vi "Material-Line1-Aquisition.vi"(8 "error in (no error)":errorcluster, 11 "Material-RunTest in":refnum<class "Material-RunTest.lvclass">) -> (0 "error out":errorcluster, 3 "Material-RunTest out":refnum<class "Material-RunTest.lvclass">)   [LabVIEW 2013, in "Material-RunTest.lvclass"]
uses:
  Material-RunTest.lvclass
  Material-RunTest.lvclass/Material-RunTest.ctl
  <instrlib>/Keyence LK-G5000/Public/enum/LKIF_OUTNO.ctl
  <userlib>/_MGI/1D Array/MGI Average/MGI Average (SGL[]).vi
  <instrlib>/Keyence LK-G5000/Keyence LK-G5000.lvlib
  Motion Control/Motion-ControlAll.lvclass
panel:
  out "Laser Value":sgl format="%_6g"
  out "Init Meas1":dbl[](array[numeric])
  out "stop collecting":bool
  out "Meas 1 Dyn Data":dbl[](graph)
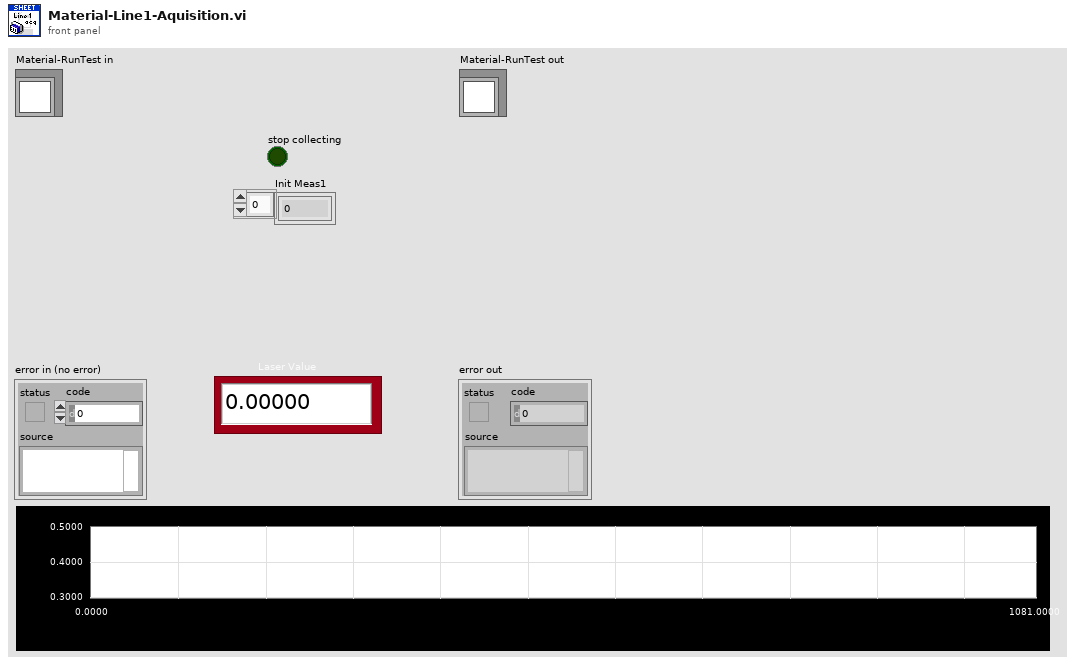
[diagram p1: front panel]
types:
  T1 = typedef "Keyence LK-G5000.lvlib/LKIF_OUTNO.ctl" = i32
  T2 = typedef "Keyence LK-G5000.lvlib/LKIF_FLOATRESULT.ctl" = i32
  T3 = cluster{"OutNo":i32, "LKIF_FLOATRESULT":T2, "Value":sgl}[]
  T4 = cluster{"OutNo":i32, "LKIF_FLOATRESULT":T2, "Value":sgl}
  T5 = cluster{waveform(dbl), waveform(dbl), waveform(dbl)}
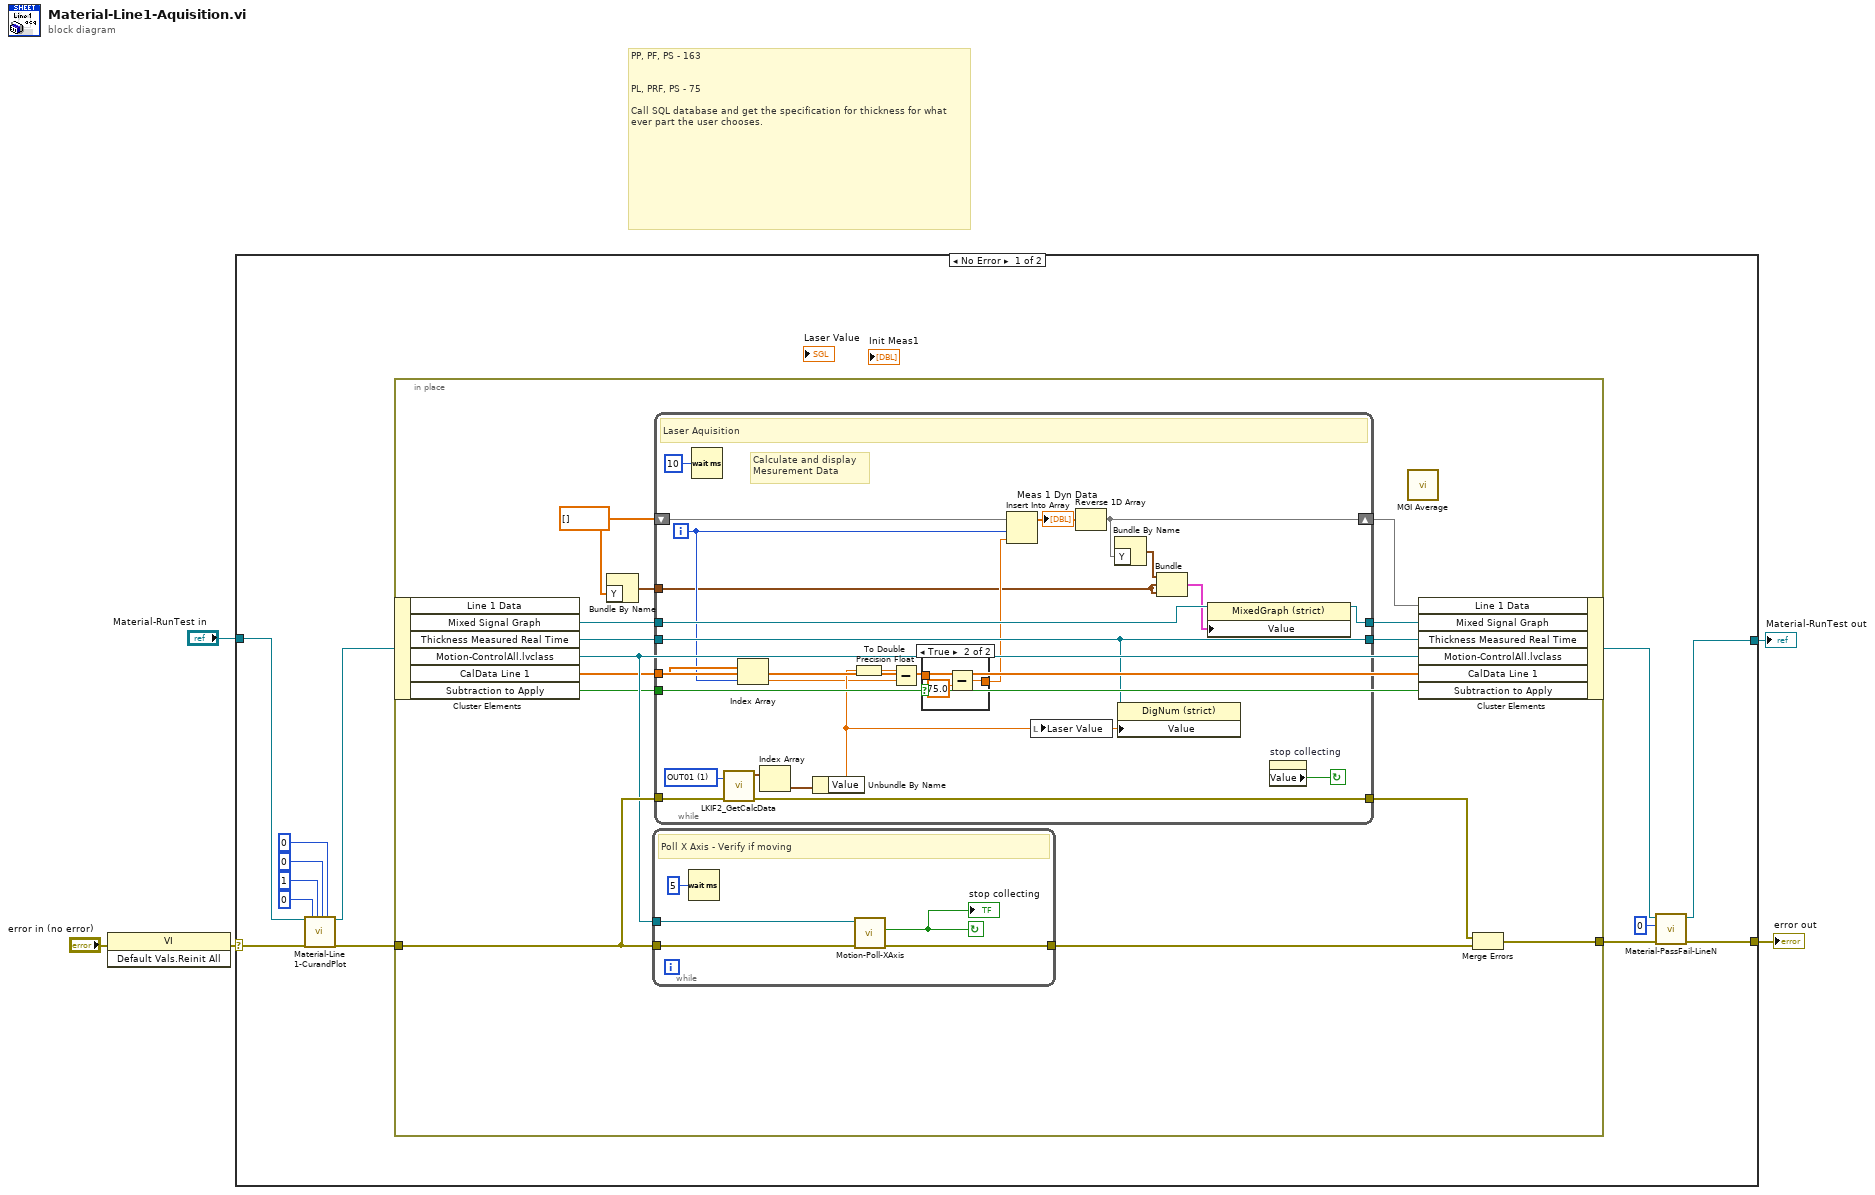
[diagram p0: block diagram]
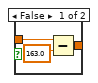
[diagram p2: hidden frame]
diagram:
  # "PP, PF, PS - 163\n\n\nPL, PRF, PS - 75\n\nCall SQL database and get the specification for thickness for what ever part the user chooses."
  n1 = invoke class="VI" method="Default Vals.Reinit All"(error in="error in (no error)") -> (error out=w1:errorcluster)  [unwired: 2 in, 2 out]
  n2 = case shown="No Error" w1 {
    selector: w1 -> [w13 w69]
    tunnel: [w6 w69] -> w5
    tunnel: [w7 w68] -> w3
    tunnel: "Material-RunTest in" -> [w18 w68]
    frame No Error {
      n3 = call "Material-Line 1-CurandPlot.vi"("Material-RunTest in"=w18, "error in (no error)"=w13, "Active Cursor Max"=u32 0, "Active Cursor Min"=u32 1, "Active Y Scale"=0, "Active Plot"=u32 0) -> ("Material-RunTest out"=w11:refnum<class "Material-RunTest.lvclass">, "error out"=w12:errorcluster)  [unwired: 12 in]
      n4 = in-place {
        in-place-border: w12 -> [w32]
        in-place-border: [w24] -> w10
        w19 = dbl[] []
        n5 = in-place-cluster #1(w11) -> ("Mixed Signal Graph"=w30:refnum<vi>, "Thickness Measured Real Time"=w31:refnum<vi>, "Motion-ControlAll.lvclass"=w27:refnum<class "Motion-ControlAll.lvclass">, "CalData Line 1"=w22:dbl[], "Subtraction to Apply"=w21:bool)  [unwired: 1 out]
        n6 = Bundle By Name("Y"=w19) -> (w20:waveform(dbl))  [unwired: 1 in]
        n7 = while {
          tunnel: w32 -> [w36]
          tunnel: [w34] -> w26
          tunnel: w27 -> [w35]
          stop <- w33 continue-if-true
          # "Poll X Axis - Verify if moving"
          n8 = Wait (ms)(milliseconds to wait=u32 5) -> ()  [unwired: 1 out]
          n9 = call "Motion-Poll-XAxis.vi"("error in (no error)"=w36, "Motion-ControlAll in"=w35) -> ("error out"=w34:errorcluster, "X axis \nstopped"=w33:bool)  [unwired: 7 in, 1 out]
          "stop collecting" <- w33
        }
        n10 = while {
          tunnel: w32 -> [w61]
          tunnel: [w57] -> w25
          tunnel: w31 -> [w47]
          shift-right: [w49] -> w23
          shift-left: w19 -> [w55]
          tunnel: w30 -> [w52]
          tunnel: [w48] -> w29
          tunnel: [w47] -> w28
          tunnel: w22 -> [w46]
          tunnel: w21 -> [w42]
          tunnel: w20 -> [w38]
          i -> [w45]
          stop <- w39 continue-if-true
          w60 = T1 1 items=["OUT01"=1, "OUT02"=2, "OUT03"=4, "OUT04"=8, "OUT05"=16, "OUT06"=32, "OUT07"=64, "OUT08"=128, "OUT09"=256, "OUT10"=512, "OUT11"=1024, "OUT12"=2048, "ALL OUT"=4095] ("OutNo (OUT1)")
          # "Calculate and display \nMesurement Data"
          # "Laser Aquisition"
          n11 = Wait (ms)(milliseconds to wait=u32 10) -> ()  [unwired: 1 out]
          n12 = call <instrlib>:"LKIF2_GetCalcData.vi"("OutNo (OUT1)"=w60, "error in (no error)"=w61) -> ("error out"=w57:errorcluster, "CalcData"=w59:T3)  [unwired: 8 in]
          n13 = Index Array(array=w46, index=w45) -> (element=w43:dbl)
          n14 = Index Array(array=w59) -> (element=w58:T4)  [unwired: 1 in]
          n15 = Unbundle By Name(w58) -> ("Value"=w54:sgl)
          n16 = To Double Precision Float(number=w54) -> (double precision float=w44:dbl)
          n17 = Subtract(x=w44, y=w43) -> (x-y=w41:dbl)
          n18 = case shown="True" w42 {
            tunnel: w41 -> [w63 w67]
            tunnel: [w62 w65] -> w40
            frame False {
              n19 = Subtract(x=w63, y=163.0) -> (x-y=w62:dbl)
            }
            frame True {
              n20 = Subtract(x=w67, y=75.0) -> (x-y=w65:dbl)
            }
          }
          n21 = Insert Into Array(array=w55, index=w45, new element=w40) -> (w53:dbl[])
          "Meas 1 Dyn Data" <- w53
          n22 = local write "Laser Value"(w54) -> ()
          n23 = Reverse 1D Array(array=w53) -> (reversed array=w49:dbl[])
          n24 = Bundle By Name("Y"=w49) -> (w50:waveform(dbl))  [unwired: 1 in]
          n25 = property class="DigNum (strict)"(reference=w47, "Value"=w54) -> ()  [unwired: 1 in, 2 out]
          n26 = Bundle(w50, w38, w38) -> (w51:T5)  [unwired: 1 in]
          n27 = property class="MixedGraph (strict)"(reference=w52, "Value"=w51) -> (reference out=w48:refnum<vi>)  [unwired: 1 in, 1 out]
          n28 = property on="stop collecting" class="Bool (strict)"() -> ("Value"=w39:bool)  [unwired: 2 in, 2 out]
        }
        n29 = call-poly <userlib>:"MGI Average.vi"() -> ()  [unwired: 2 in, 1 out]
        n30 = in-place-cluster #1("Line 1 Data"=w23, "Mixed Signal Graph"=w29, "Thickness Measured Real Time"=w28, "Motion-ControlAll.lvclass"=w27, "CalData Line 1"=w22, "Subtraction to Apply"=w21) -> (w9:refnum<class "Material-RunTest.lvclass">)
        n31 = Merge Errors(w25, w26) -> (w24:errorcluster)
      }
      n32 = call "Material-PassFail-LineN.vi"("error in (no error)"=w10, "Line?"=0, "Material-RunTest in"=w9) -> ("error out"=w6:errorcluster, "Material-RunTest out"=w7:refnum<class "Material-RunTest.lvclass">)  [unwired: 7 in]
    }
    frame Error {
    }
  }
  "error out" <- w5
  "Material-RunTest out" <- w3
